vi "bindata subset by kwarg_name.vi"(8 "error in (no error)":errorcluster, 10 "kwarg_name":string, 11 "Bindata & descr in":T1) -> (0 "error out":errorcluster, 2 "bindata descr":T2, 3 "bindata":u8[](array[numeric]))   [LabVIEW 2018, in "LV-Julia_ZMQ-Roundtrip_lib.lvlib"]
uses:
  LV-Julia_ZMQ-Roundtrip_lib.lvlib
  Bindata description.ctl
  Bindata&description.ctl
  <vilib>/Utility/error.llb/Error Cluster From Error Code.vi
  <vilib>/ErrorRing/Error Ring.xnode
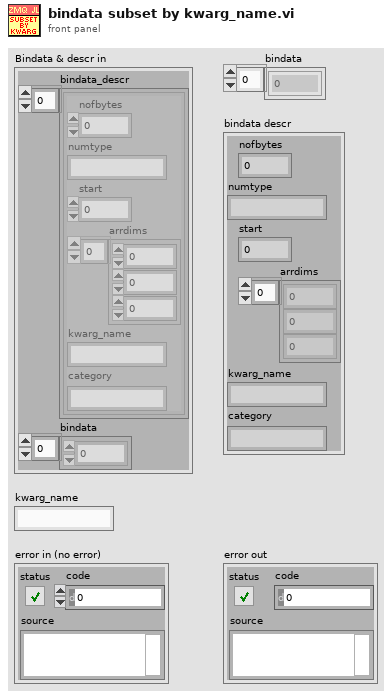
[diagram p1: front panel]
types:
  T1 = typedef "Bindata&description.ctl" = cluster{"bindata_descr":T2[], "bindata":u8[]}
  T2 = typedef "LV-Julia_ZMQ-Roundtrip_lib.lvlib/Bindata description.ctl" = cluster{"nofbytes":i32, "numtype":string, "start":i32, "arrdims":i32[], "kwarg_name":string, "category":string}
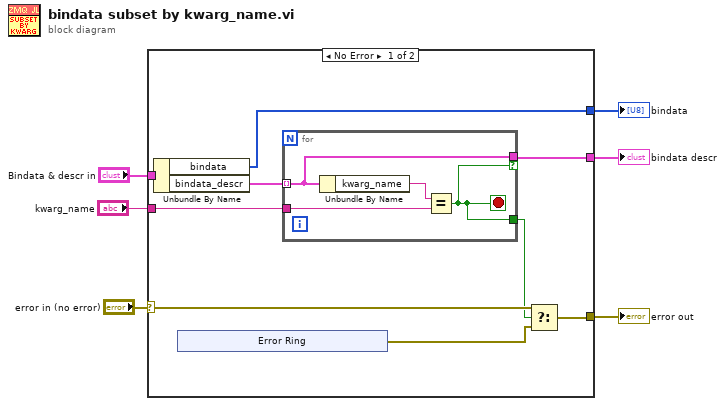
[diagram p0: block diagram]
diagram:
  n1 = case shown="No Error" "error in (no error)" {
    selector: "error in (no error)" -> [w9 w25]
    tunnel: [w15 _] -> w6
    tunnel: "Bindata & descr in" -> [w14 _]
    tunnel: "kwarg_name" -> [w12 _]
    tunnel: [w11 _] -> w3
    tunnel: [w10 w25] -> w2
    frame No Error {
      n2 = Unbundle By Name(w14) -> ("bindata"=w15:u8[], "bindata_descr"=w13:T2[])
      n3 = xnode "Error Ring"() -> ("error out"=w7:errorcluster)
      n4 = for {
        tunnel: w13 -> [w22] mode=indexing
        tunnel: w12 -> [w23]
        tunnel: [w22] -> w11 if=w21
        tunnel: [w21] -> w8
        stop <- w21 stop-if-true
        n5 = Unbundle By Name(w22) -> ("kwarg_name"=w24:string)
        n6 = Equal?(x=w24, y=w23) -> (x = y?=w21:bool)
      }
      n7 = Select(t=w9, s=w8, f=w7) -> (s? t:f=w10:errorcluster)
    }
    frame Error {
    }
  }
  "error out" <- w2
  "bindata" <- w6
  "bindata descr" <- w3
